vi "Test Client.vi"() -> ()   [LabVIEW 2013]
uses:
  <vilib>/httpClient/POSTBuffer.vi
  <vilib>/httpClient/LabVIEWHTTPClient.lvlib
panel:
  out "body":string
  out "headers":string
  in  "Configuration":string="Cat=General\nTag=e:c2tc16\nType=float\nLo=17\nHi=28\nDesc=Hall%20temperature%20west%20wall%20thermocouple\n=\nCat=General\nTag=d:outtmp\nType=float\nLo=0\nHi=100\nDesc=Outside%20temperature\n=\nCat=General\nTag=l:lgtemp\nType=float\nLo=65\nHi=85\nDesc=Linac%20Gallery%20temperature\n=\nCat=General\nTag=l:lghum\nType=float\nLo=20\nHi=80\nDesc=Linac%20Gallery%20humidity\n=\nCat=Cryo\nTag=e:mclln2\nLo=35\nHi=75\nDesc=Solenoid%20LN2%20level\n=\nCat=Cryo\nTag=e:mcllhe\nLo=36\nHi=46\nDesc=Solenoid%20LHe%20level\n=\nCat=Solenoid\nTag=e:mcsoli\nDesc=Solenoid%20current\n=\nCat=Solenoid\nTag=e:mcsolv\nDesc=Solenoid%20ps%20voltage\n=\nCat=Solenoid\nTag=e:mctdhe\nLo=3.6\nHi=4.5\nDesc=Solenoid%20LHe%20temperature\n=\nCat=Radiation\nTag=e:mtamr1\nType=float\nLo=0\nHi=10\nDesc=IC1%20dose%20rate%2060s\n=\nCat=Radiation\nTag=e:mtamr2\nType=float\nLo=0\nHi=40\nDesc=IC2%20dose%20rate%2060s\n=\nCat=Radiation\nTag=e:mtamr3\nType=float\nLo=0\nHi=24\nDesc=IC3%20dose%20rate%2060s\n=\nCat=Radiation\nTag=e:mtamr4\nType=float\nLo=0\nHi=12\nDesc=IC4%20dose%20rate%2060s\n=\nCat=Radiation\nTag=g:rd2043\nType=float\nLo=0\nHi=10\nDesc=Chipmunk%20dose%20rate%2060s\n=\nCat=RF201\nTag=l:ipa17f\nType=float\nLo=100\nDesc=IPA1%20fwd%20power\n=\nCat=RF201\nTag=l:ipa17r\nType=float\nHi=72\nDesc=IPA1%20ref%20power\n=\nCat=RF201\nTag=l:ipa27f\nType=float\nLo=2\nDesc=IPA2%20fwd%20power\n=\nCat=RF201\nTag=l:ipa27r\nType=float\nHi=0.125\nDesc=IPA2%20ref%20power\n=\nCat=RF201\nTag=l:dr7f\nType=float\nLo=100\nDesc=Driver%20fwd%20power\n=\nCat=RF201\nTag=l:dr7r\nType=float\nHi=10.5\nDesc=Driver%20ref%20power\n=\nCat=RF201\nTag=l:dr7sv\nType=float\nLo=400\nDesc=Driver%20screen%20voltage\n=\nCat=RF201\nTag=l:rf7hv\nType=float\nLo=33\nHi=42\nDesc=Modulator%20HV\n=\nCat=RF201\nTag=l:md7ov\nType=float\nDesc=Modulator%20output%20voltage\n=\nCat=RF201\nTag=l:md7oi\nType=float\nDesc=Modulator%20output%20current\n=\nCat=RF201\nTag=l:rf7pav\nType=float\nDesc=7835%20filament%20voltage\n=\nCat=RF201\nTag=l:rf7pai\nType=float\nLo=6500\nHi=7350\nDesc=7835%20filament%20current\n=\nCat=RF201\nTag=l:pa7ion\nType=float\nDesc=7835%20filament%20IP%20current\nHi=0.1\n=\nCat=MICECavity\nTag=e:201vac\nType=float\nLo=1E-8\nHi=1E-6\nDesc=Cavity%20top%20vacuum%20IG\n=\nCat=MICECavity\nTag=e:c2ctpr\nType=float\nLo=1E-8\nHi=3E-6\nDesc=Cavity%20top%20vacuum%20CCG\n=\nCat=MICECavity\nTag=e:c2cbig\nLo=1E-8\nHi=1E-6\nDesc=Cavity%20bot%20vacuum%20IG\n=\nCat=MICECavity\nTag=e:c2frg1\nLo=1E-8\nHi=1E-6\nDesc=Cavity%20bot%20vacuum%20FRG\n=\nCat=MICECavity\nTag=e:solig2\nType=float\nLo=1E-8\nHi=1E-6\nDesc=Vessel%20vacuum%20IG\n=\nCat=MICECavity\nTag=e:c2cbpr\nType=float\nLo=1E-8\nHi=1E-6\nDesc=Vessel%20vacuum%20CCG\n=\nCat=MICECavity\nTag=e:c2clig\nType=float\nDesc=Left%20coupler%20vacuum%20IG\n=\nCat=MICECavity\nTag=e:c2crig\nType=float\nDesc=Right%20coupler%20vacuum%20IG\n=\nCat=MICECavity\nTag=e:c2clpr\nType=float\nLo=1E-7\nHi=1.2E-6\nDesc=Left%20coupler%20vacuum%20CCG\n=\nCat=MICECavity\nTag=e:c2crpr\nType=float\nLo=1E-7\nHi=1E-6\nDesc=Right%20coupler%20vacuum%20CCG\n=\nCat=MICECavity\nTag=e:c2frg2\nLo=1E-9\nHi=1E-6\nDesc=Getter%20manifold%20vacuum%20IG\n=\nCat=MICECavity\nTag=e:c2wmig\nType=float\nLo=1E-8\nHi=1E-7\nDesc=Wall%20manifold%20vacuum%20IG\n=\nCat=MICECavity\nTag=e:mccwou\nType=float\nLo=0\nHi=110\nDesc=Chiller%20input%20return%20pressure\n=\nCat=MICECavity\nTag=e:mccwin\nType=float\nLo=45\nHi=80\nDesc=Chiller%20output%20supply%20pressure\n=\nCat=MICECavity\nTag=e:c2wmsp\nType=float\nLo=30\nHi=80\nDesc=Hall%20water%20supply%20pressure\n=\nCat=MICECavity\nTag=e:c2cvsp\nType=float\nLo=20\nHi=80\nDesc=Cavity%20body%20water%20supply%20pressure\n=\nCat=MICECavity\nTag=e:c2cpsp\nType=float\nLo=20\nHi=80\nDesc=Coupler%20water%20supply%20pressure\n=\nCat=MICECavity\nTag=e:c2cprp\nType=float\nLo=0\nHi=30\nDesc=Coupler%20water%20return%20pressure\n=\nCat=MICECavity\nTag=e:c2cvrp\nType=float\nLo=0\nHi=30\nDesc=Cavity%20body%20water%20return%20pressure\n=\nCat=MICECavity\nTag=e:c2wmrp\nType=float\nLo=0\nHi=30\nDesc=Hall%20water%20return%20pressure\n=\nCat=MICECavity\nTag=e:c2wmst\nType=float\nLo=10\nHi=40\nDesc=Hall%20water%20supply%20temperature\n=\nCat=MICECavity\nTag=e:c2cvst\nType=float\nLo=10\nHi=40\nDesc=Cavity%20body%20water%20supply%20temperature\n=\nCat=MICECavity\nTag=e:c2clst\nType=float\nLo=10\nHi=40\nDesc=Left%20coupler%20water%20supply%20temperature\n=\nCat=MICECavity\nTag=e:c2crst\nType=float\nLo=10\nHi=40\nDesc=Right%20coupler%20water%20supply%20temperature\n=\nCat=MICECavity\nTag=e:c2cvrt\nType=float\nLo=10\nHi=40\nDesc=Cavity%20body%20water%20return%20temperature\n=\nCat=MICECavity\nTag=e:c2clrt\nType=float\nLo=10\nHi=40\nDesc=Left%20coupler%20water%20return%20temperature\n=\nCat=MICECavity\nTag=e:c2crrt\nType=float\nLo=10\nHi=40\nDesc=Right%20coupler%20water%20return%20temperature\n=\nCat=MICECavity\nTag=e:c2wmrt\nType=float\nLo=10\nHi=40\nDesc=Hall%20water%20return%20temperature\n=\nCat=MICECavity\nTag=e:c2fl01\nType=float\nLo=0.8\nHi=1.2\nDesc=Coupler%20water%20flow\n=\nCat=MICECavity\nTag=e:c2fl03\nType=float\nLo=0.8\nHi=1.2\nDesc=Cavity%20body%20water%20flow\n=\nCat=MICECavity\nTag=e:c2tc\nType=float\nLo=17\nHi=25\nDesc=Cavity%20avg%20temperature\n=\nCat=MICECavity\nTag=e:c2dtc\nType=float\nLo=-4.5\nHi=0.5\nDesc=Cavity%20temperature%20differential\n=\nCat=MICECavity\nTag=e:c2tcus\nType=float\nLo=17\nHi=22.5\nDesc=Cavity%20upstream%20face%20temperature\n=\nCat=MICECavity\nTag=e:c2tcds\nType=float\nLo=17\nHi=26.5\nDesc=Cavity%20downstream%20face%20temperature\n=\nCat=MICECavity\nTag=e:c2tc01\nType=float\nLo=17\nHi=23\nDesc=Cavity%20us%20tc%201\n=\nCat=MICECavity\nTag=e:c2tc02\nType=float\nLo=17\nHi=23\nDesc=Cavity%20us%20tc%202\n=\nCat=MICECavity\nTag=e:c2tc03\nType=float\nLo=17\nHi=23\nDesc=Cavity%20us%20tc%203\n=\nCat=MICECavity\nTag=e:c2tc04\nType=float\nLo=17\nHi=23\nDesc=Cavity%20us%20tc%204\n=\nCat=MICECavity\nTag=e:c2tc05\nType=float\nLo=17\nHi=23\nDesc=Cavity%20us%20tc%205\n=\nCat=MICECavity\nTag=e:c2tc06\nType=float\nLo=17\nHi=23\nDesc=Cavity%20us%20tc%206\n=\nCat=MICECavity\nTag=e:c2tc09\nType=float\nLo=17\nHi=27\nDesc=Cavity%20ds%20tc%201\n=\nCat=MICECavity\nTag=e:c2tc10\nType=float\nLo=17\nHi=27\nDesc=Cavity%20ds%20tc%202\n=\nCat=MICECavity\nTag=e:c2tc11\nType=float\nLo=17\nHi=27\nDesc=Cavity%20ds%20tc%203\n=\nCat=MICECavity\nTag=e:c2tc12\nType=float\nLo=17\nHi=27\nDesc=Cavity%20ds%20tc%204\n=\nCat=MICECavity\nTag=e:c2tc13\nType=float\nLo=17\nHi=27\nDesc=Cavity%20ds%20tc%205\n=\nCat=MICECavity\nTag=e:c2tc14\nType=float\nLo=17\nHi=27\nDesc=Cavity%20ds%20tc%206\n=\nCat=MICECavity\nTag=e:c2tc07\nType=float\nLo=16\nHi=28\nDesc=Vessel us flange plate tc\n=\nCat=MICECavity\nTag=e:c2tc08\nType=float\nLo=16\nHi=28\nDesc=Vessel%20center%20ring%20tc\n=\nCat=MICECavity\nTag=e:c2tc15\nType=float\nLo=17\nHi=28\nDesc=Vessel%20ds%20flange%20plate%20tc\n=\nCat=MICECavity\nTag=e:c2ach4\nType=float\nLo=30\nHi=35\nDesc=Coax%20gas%20pressure\n=\nCat=MICECavity\nTag=e:c2apr1\nType=float\nLo=-10\nHi=90\nDesc=Tuner%20actuator%20input%20pressure\n=\nCat=MICECavity\nTag=e:c2apr2\nType=float\nLo=-1\nHi=20\nDesc=Tuner%20actuator%20push%20pressure\n=\nCat=MICECavity\nTag=e:c2apr3\nType=float\nLo=-1\nHi=20\nDesc=Tuner%20actuator%20pull%20pressure\n=\nCat=MICECavity\nTag=e:c2vpr2\nType=float\nLo=-1\nHi=20\nDesc=Tuner%20actuator%20push%20pressure\n=\nCat=MICECavity\nTag=e:c2vpr3\nType=float\nLo=-1\nHi=20\nDesc=Tuner%20actuator%20pull%20pressure\n=\nCat=MICECavity\nTag=e:c2ampl\nType=float\nDesc=Signal%20generator%20drive%20level\n=\nCat=MICECavity\nTag=e:c2prob\nType=float\nLo=0.02\nHi=1.65\nDesc=Cavity%20pickup%20envelope%20peak\n=\nCat=MICECavity\nTag=e:c2freq\nType=float\nLo=0.81\nHi=1.25\nDesc=Cavity%20frequency%20-%20200%20MHz\n=\nCat=MICECavity\nTag=e:c2phas\nType=float\nDesc=Cavity%20phase\nLo=-1\nHi=1\n=\nCat=MICECavity\nTag=e:c2rtio\nType=float\nDesc=Cavity%20pickup-to-reflected%20ratio%20left\n=\nCat=MICECavity\nTag=e:c2rtir\nType=float\nDesc=Cavity%20pickup-to-reflected%20ratio%20right\n=\nCat=MICECavity\nTag=e:c2puls\nType=int\nDesc=Number%20of%20RF%20pulses\n=\nCat=MICECavity\nTag=e:c2sprk\nType=int\nDelta=1\nDesc=Number%20of%20sparks\n=\nCat=MICECavity\nTag=e:c2sptm\nType=int\nDesc=Pulses%20since%20last%20spark\n=\nCat=MICECavity\nTag=e:c2prsk\nType=float\nDesc=Pickup%20peak%20at%20last%20spark\n=\n"
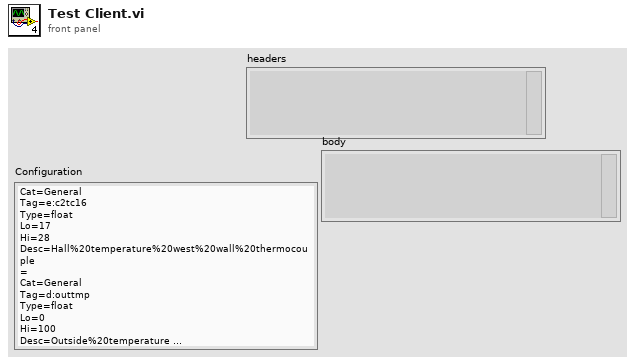
[diagram p1: front panel]
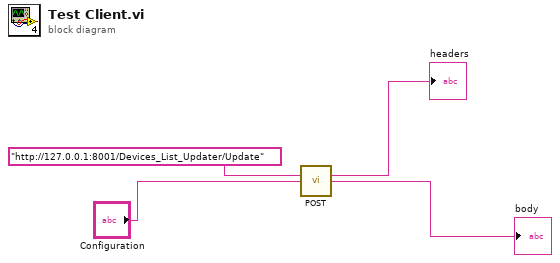
[diagram p0: block diagram]
diagram:
  n1 = call-poly <vilib>:"POST.vi"("url"="http://127.0.0.1:8001/Devices_List_Updater/Update", "buffer"="Configuration") -> ("headers"=→"headers":string, "body"=→"body":string)  [unwired: 10 in, 2 out]
